vi "fgv_reg-test_config.vi"(7 "cmd":T2, 11 "TestConfig":T1) -> (3 "TestConfig out":T1)   [LabVIEW 2019]
uses:
  _ctrl/rw.ctl
  Setting_reg.ctl
panel:
  # "Highpower"
  # "Control"
  # "Highpower"
  # "Control"
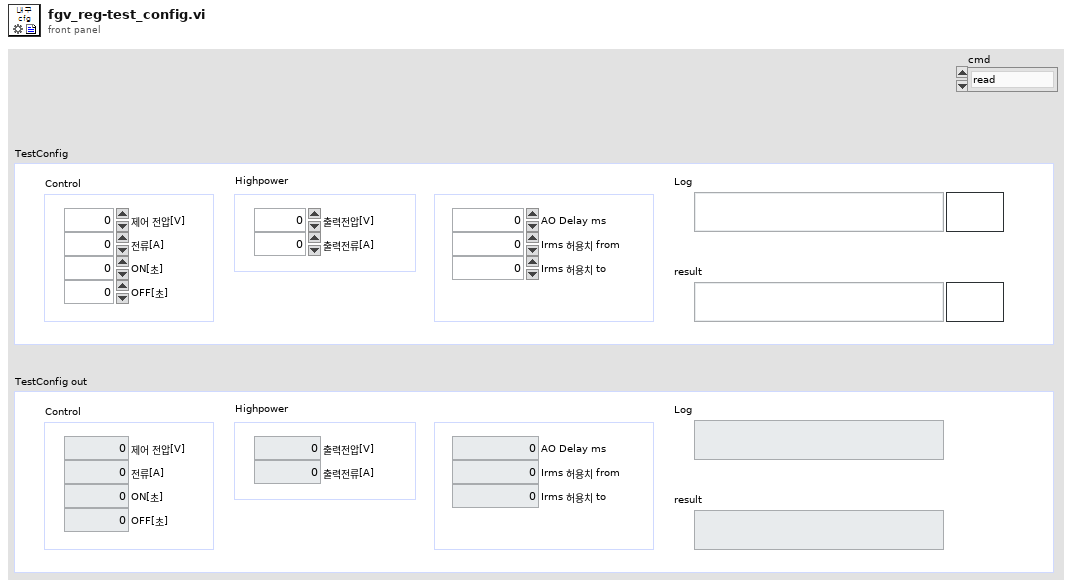
[diagram p1: front panel]
types:
  T1 = typedef "Setting_reg.ctl" = cluster{"제어 전압[V]":dbl, "출력전압[V]":dbl, "전류[A]":dbl, "출력전류[A]":dbl, "ON[초]":dbl, "OFF[초]":dbl, "Irms 허용치 from ":dbl, "Irms 허용치 to":dbl, "AO Delay ms":u32, "Log":path, "result":path}
  T2 = typedef "rw.ctl" = enum16{"read", "write"}
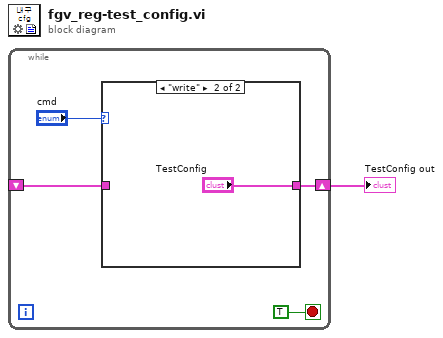
[diagram p0: block diagram]
diagram:
  n1 = while {
    shift-right: [w3] -> w1
    shift-left: _ -> [w2]
    stop <- TRUE stop-if-true
    n2 = case shown="\"write\"" "cmd" {
      tunnel: [w6 "TestConfig"] -> w3
      tunnel: w2 -> [w6 _]
      frame "read", Default {
      }
      frame "write" {
      }
    }
  }
  "TestConfig out" <- w1
